vi "FTW-Connector-SpawnNewActor-Core.vi"(0 "FTW Actor Connector Type":refnum<class "FTW-ActorConnector.lvclass">, 5 "Configuration":string="{\n  \"Identity\": \"ActorName\",\n  \"DebugEnableInboxLogging\": false,\n  \"DebugEnableJobLogging\": false,\n  \"InboxAddress\": \"inproc://*\",\n  \"DebugShowPanel\": false\n}", 11 "error in":errorcluster) -> (4 "FTW Actor Connector":refnum<class "FTW-ActorConnector.lvclass">, 6 "Initialized Response":string, 8 "Instance Inbox Address":string, 15 "error out":errorcluster)   [LabVIEW 2015, in "FTW-ActorConnector.lvclass"]
uses:
  FTW-ActorConnector.lvclass
  JSON/core/FTW-JSON-Core-EncodingFlags.vi
  JSON/FTW-JSON-Parse.vi
  Reflection/FTW-Reflection-Type.vi
  CodeGen/JSON Deserialize/FTW-JSON-Core-GetFlattenedValue.vi
  CodeGen/JSON Deserialize/FTW-JSON-Deserialize.xnode
  Endpoint/FTW-Endpoint.lvclass
  Ether/FTW-Ether.lvclass
panel:
  # "Inputs"
  # "Outputs"
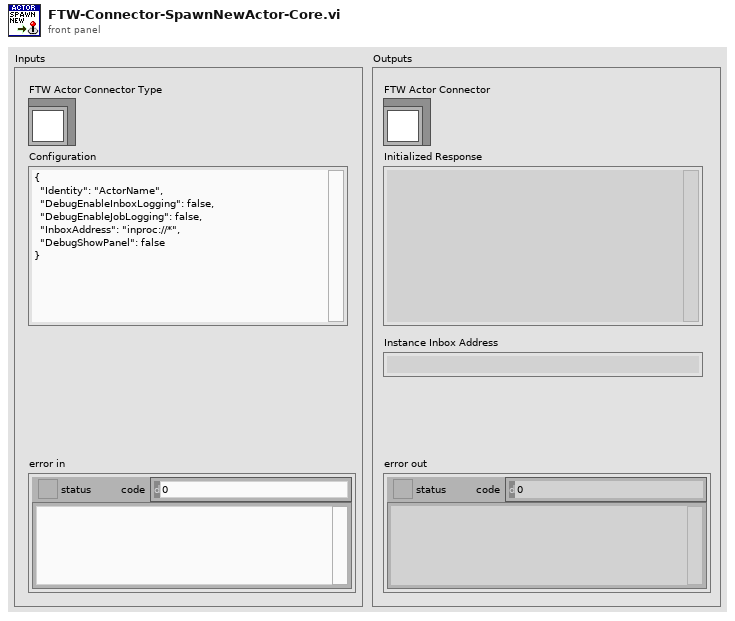
[diagram p1: front panel]
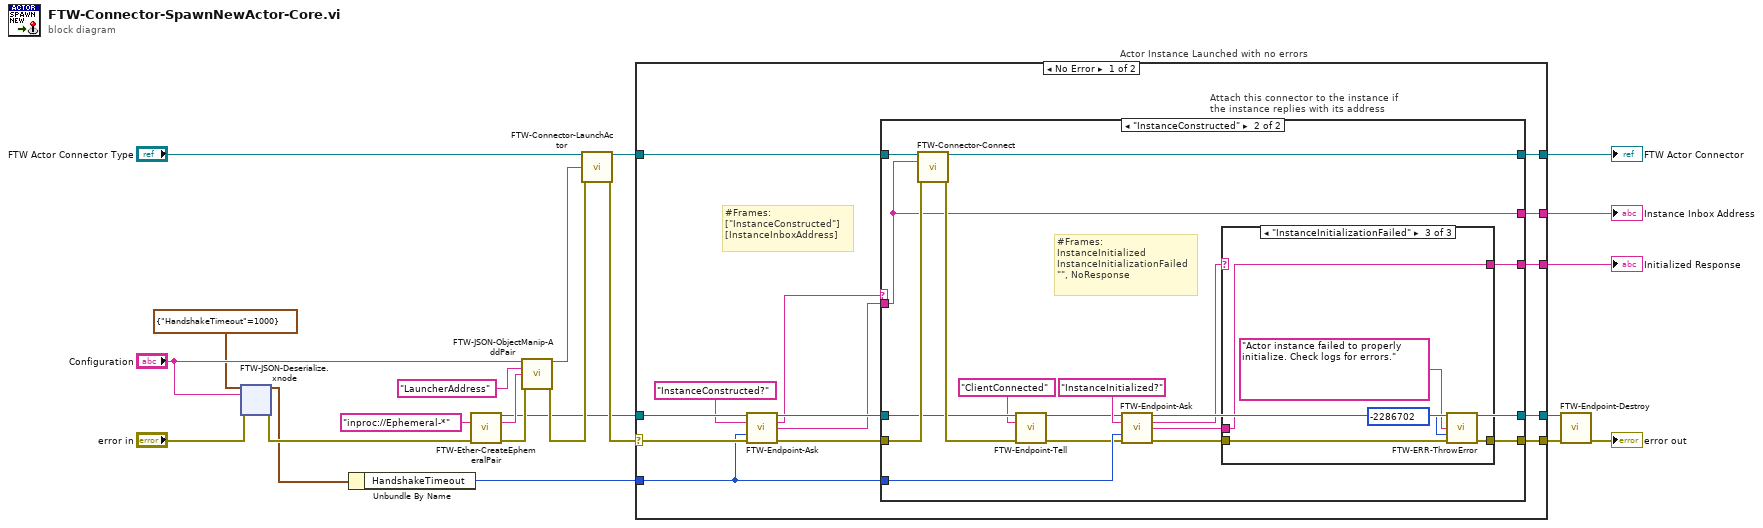
[diagram p0: block diagram]
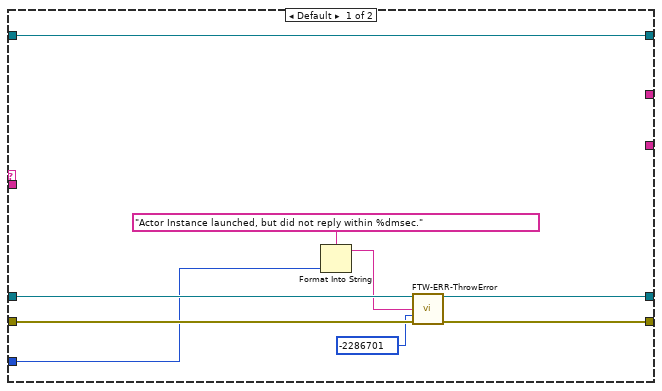
[diagram p2: hidden frame]
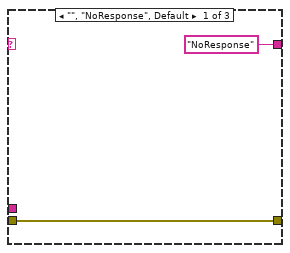
[diagram p3: hidden frame]
diagram:
  n1 = xnode "FTW-JSON-Deserialize.xnode"("Type and Defaults"=cluster{"HandshakeTimeout":i32} {"HandshakeTimeout"=1000}, "JSON String"="Configuration", "error in"="error in") -> ("Values"=w3:cluster{"HandshakeTimeout":i32}, "error out"=w22:errorcluster)
  n2 = Unbundle By Name(w3) -> ("HandshakeTimeout"=w2:i32)
  n3 = call "FTW-Ether-CreateEphemeralPair.vi"("Requested Ephemeral Address"="inproc://Ephemeral-*", "error in"=w22) -> ("Ephemeral Endpoint"=w6:refnum<class "FTW-Endpoint.lvclass">, "Actual Ephemeral Address"=w10:string, "error out"=w9:errorcluster)  [unwired: 11 in]
  n4 = call "FTW-JSON-ObjectManip-AddPair.vi"("Input JSON Object"="Configuration", "Key"="LauncherAddress", "Value"=w10, "error in"=w9) -> ("Output JSON Object"=w8:string, "error out"=w12:errorcluster)  [unwired: 10 in]
  n5 = call-dynamic "FTW-Connector-LaunchActor.vi"("FTW Actor Connector Type"="FTW Actor Connector Type", "Configuration"=w8, "error in"=w12) -> ("FTW Actor Connector"=w13:refnum<class "FTW-ActorConnector.lvclass">, "error out"=w11:errorcluster)  [unwired: 11 in]
  n6 = case "Actor Instance Launched with no errors" shown="No Error" w11 {
    selector: w11 -> [w31 w72]
    tunnel: [w36 w72] -> w14
    tunnel: w13 -> [w35 w73]
    tunnel: [w34 w73] -> w20
    tunnel: w6 -> [w32 w71]
    tunnel: w2 -> [w30 _]
    tunnel: [w33 w71] -> w15
    tunnel: [w27 _] -> w18
    tunnel: [w26 _] -> w17
    frame No Error {
      # "#Frames:\n[\"InstanceConstructed\"]\n[InstanceInboxAddress]"
      n7 = call-dynamic "FTW-Endpoint-Ask.vi"("FTW Endpoint"=w32, "Request Header"="InstanceConstructed?" ("Header"), "Timeout"=w30, "error in"=w31) -> ("FTW Endpoint out"=w28:refnum<class "FTW-Endpoint.lvclass">, "Response Header"=w24:string, "Response Body"=w23:string, "error out"=w29:errorcluster)  [unwired: 5 in, 3 out]
      n8 = case "Attach this connector to the instance if\nthe instance replies with its address" shown="\"InstanceConstructed\"" w24 {
        tunnel: [w42 w47] -> w36
        tunnel: w35 -> [w44 w59]
        tunnel: [w44 w58] -> w34
        tunnel: w28 -> [w41 w53]
        tunnel: w29 -> [w43 w60]
        tunnel: [w41 w57] -> w33
        tunnel: w30 -> [w39 w55]
        tunnel: w23 -> [_ w54]
        tunnel: [_ w48] -> w27
        tunnel: [_ w54] -> w26
        frame Default {
          n9 = Format Into String(format string="Actor Instance launched, but did not reply within %dmsec." ("Error Message"), w39) -> (resulting string=w38:string)  [unwired: 2 in, 1 out]
          n10 = call "FTW-ERR-ThrowError.vi"("Error Message"=w38, "Error Code"=-2286701, "error in"=w43) -> ("error out"=w42:errorcluster)  [unwired: 12 in]
        }
        frame "InstanceConstructed" {
          # "#Frames:\nInstanceInitialized\nInstanceInitializationFailed\n\"\", NoResponse"
          n11 = call-dynamic "FTW-Connector-Connect.vi"("FTW Actor Connector Type"=w59, "Instance Inbox Address"=w54, "error in"=w60) -> ("FTW Actor Connector"=w58:refnum<class "FTW-ActorConnector.lvclass">, "error out"=w61:errorcluster)  [unwired: 11 in]
          n12 = call-dynamic "FTW-Endpoint-Tell.vi"("FTW Endpoint"=w53, "Message Header"="ClientConnected", "error in"=w61) -> ("FTW Endpoint out"=w52:refnum<class "FTW-Endpoint.lvclass">, "error out"=w51:errorcluster)  [unwired: 10 in, 1 out]
          n13 = call-dynamic "FTW-Endpoint-Ask.vi"("FTW Endpoint"=w52, "Request Header"="InstanceInitialized?", "Timeout"=w55, "error in"=w51) -> ("FTW Endpoint out"=w57:refnum<class "FTW-Endpoint.lvclass">, "Response Header"=w49:string, "Response Body"=w45:string, "error out"=w46:errorcluster)  [unwired: 5 in, 3 out]
          n14 = case shown="\"InstanceInitializationFailed\"" w49 {
            tunnel: ["NoResponse" ("f") w64 w66] -> w48
            tunnel: [w62 w65 w69] -> w47
            tunnel: w46 -> [w62 w65 w70]
            tunnel: w45 -> [_ w64 w66]
            frame "", "NoResponse", Default {
            }
            frame "InstanceInitialized" {
            }
            frame "InstanceInitializationFailed" {
              n15 = call "FTW-ERR-ThrowError.vi"("Error Message"="Actor instance failed to properly initialize. Check logs for errors.", "Error Code"=-2286702, "error in"=w70) -> ("error out"=w69:errorcluster)  [unwired: 12 in]
            }
          }
        }
      }
    }
    frame Error {
    }
  }
  "FTW Actor Connector" <- w20
  "Initialized Response" <- w18
  "Instance Inbox Address" <- w17
  n16 = call-dynamic "FTW-Endpoint-Destroy.vi"("FTW Endpoint"=w15, "error in"=w14) -> ("error out"=→"error out":errorcluster)  [unwired: 13 in]
